vi "Test_RegisterForWrongType_Listbox_Error.vi"(8 "error in (no error)":errorcluster, 11 "TestActorEvents In":refnum<class "TestActorEvents.lvclass">) -> (0 "error out":errorcluster, 3 "TestActorEvents Out":refnum<class "TestActorEvents.lvclass">)   [LabVIEW 2017, in "TestActorEvents.lvlib" / "TestActorEvents.lvclass"]
uses:
  TestActorEvents.lvclass
  IViewModel/IViewModel/IViewModel.lvclass
  C:/Git/mva-framework/Framework/IViewManager/IViewManager/IViewManager.lvclass
  C:/Program Files (x86)/National Instruments/LabVIEW 2017/vi.lib/ActorFramework/Actor/Actor.lvclass
  ViewableListboxBadReg/ViewableListboxBadReg.lvclass
  C:/Git/mva-framework/_Test/Doubles/ViewableDoubles/LeakyViewable/LeakyViewable.lvclass
  C:/Git/mva-framework/Framework/IViewable/IViewable/IViewable.lvclass
  IModel/IModel/IModel.lvclass
  Mediator/Mediator/Mediator.lvclass
  C:/Git/mva-framework/Framework/IMediator/IMediator/IMediator.lvclass
  _Test/Doubles/ViewableDoubles/LeakyViewable/Leak Location.ctl
  _Test/Doubles/ViewableDoubles/LeakyViewable/LeakyViewable.lvclass/LeakyViewable.ctl
  IViewModel/IViewModel/IViewModel.lvclass/IViewModel.ctl
  IViewManager/IViewManager Messages/Launch Nested Views Msg/Launch Nested Views Msg.lvclass/Launch Nested Views Msg.ctl
  IViewManager/IViewManager/IViewManager.lvclass/IViewManager.ctl
  <vilib>/ActorFramework/Message Enqueuer/Message Enqueuer.lvclass/Message Enqueuer.ctl
  IViewManager/IViewManager Messages/Launch Nested Views Msg/Pack Launch Nested Views Msg.vi
  IViewManager/IViewManager/Write Startup Launch Nested Views Msg.vi
  <vilib>/ActorFramework/Message Enqueuer/Enqueue.vi
  <vilib>/ActorFramework/Stop Msg/Stop Msg.lvclass
  C:/Program Files (x86)/National Instruments/LabVIEW 2017/vi.lib/ActorFramework/Message/Message.lvclass
  <vilib>/ActorFramework/Message Priority Queue/Priority Enqueue.vi
  IViewable/IViewable/IViewable.lvclass
  IViewable/IApplicationStyle/IApplicationStyle.lvclass
  IViewManager/IViewManager Messages/Launch Nested Views Msg/Launch Nested Views Msg.lvclass
  <vilib>/addons/_JKI Toolkits/VI Tester/TestCase.llb/TestCase.lvclass
  <vilib>/ActorFramework/Actor/Actor.lvclass
  _Test/Doubles/ViewableDoubles/LeakyViewable/LeakyViewable.lvclass
  C:/Program Files (x86)/National Instruments/LabVIEW 2017/vi.lib/addons/_JKI Toolkits/VI Tester/TestCase.llb/TestCase.lvclass
panel:
  out "Error Status":errorcluster
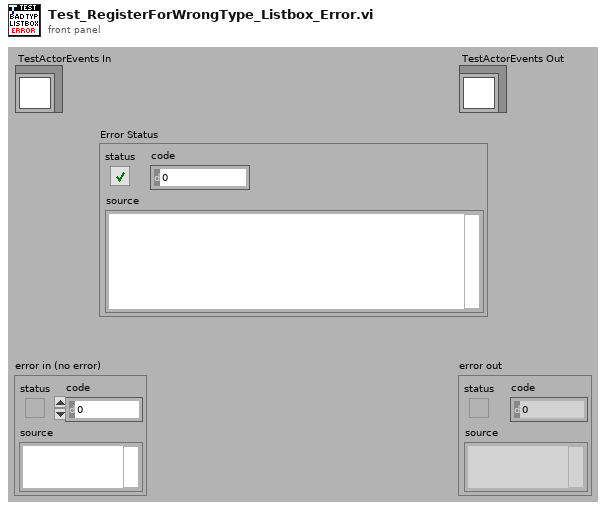
[diagram p1: front panel]
types:
  T1 = typedef "ViewableDoubles.lvlib/LeakyViewable.lvclass/Leak Location.ctl" = enum16{"Pre Launch Init", "Entering Actor Core", "Actor Core", "Exiting Actor Core", "Stop Core", "Handle Error"}
  T2 = cluster{"Location":T1, "State":refnum<class "IViewable.lvclass">, "Error Status":errorcluster}
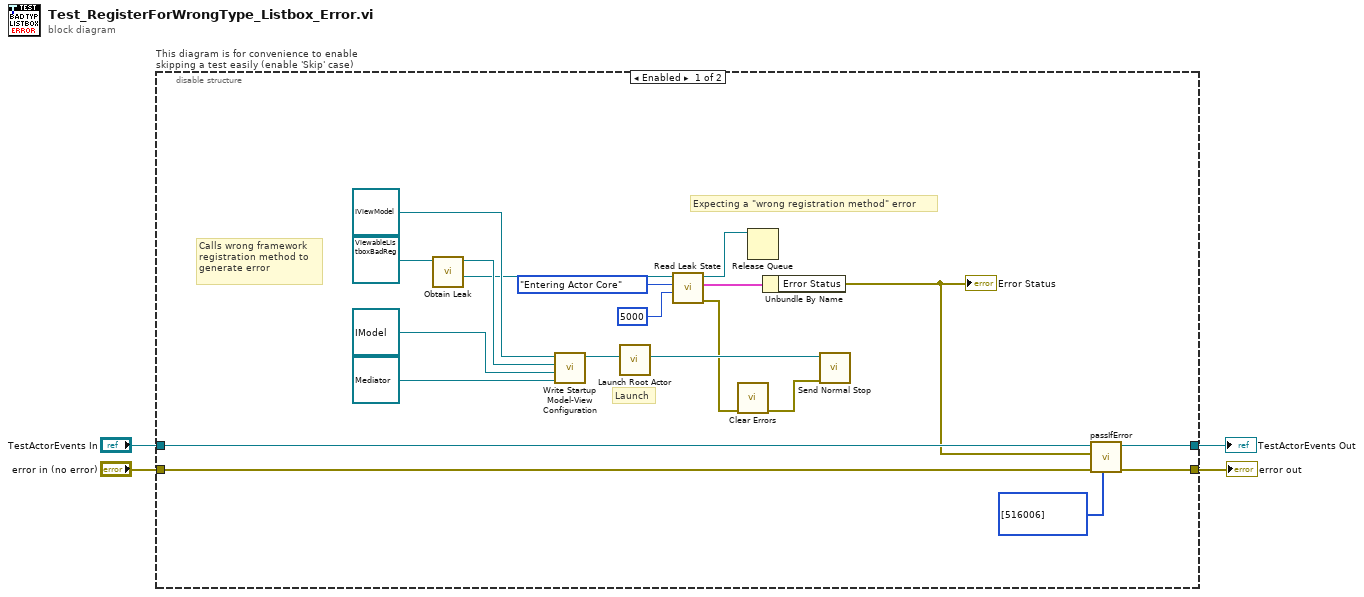
[diagram p0: block diagram]
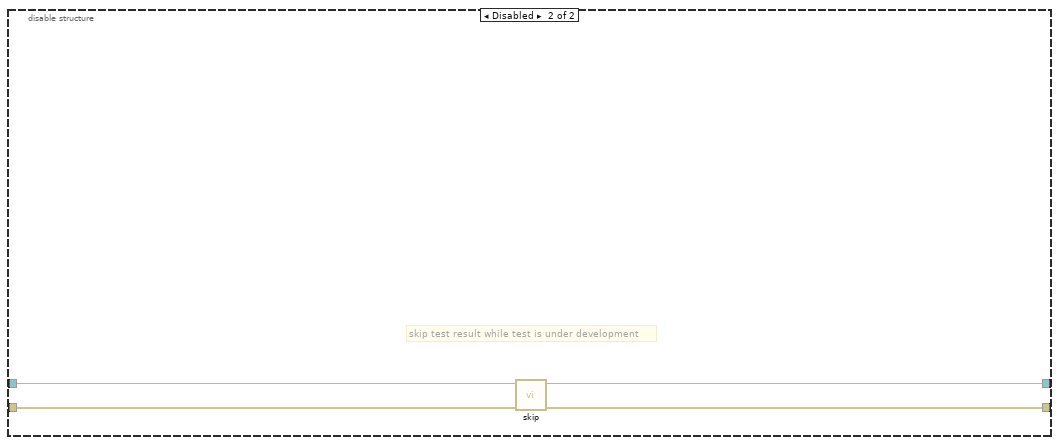
[diagram p2: hidden frame]
diagram:
  n1 = disable-structure "This diagram is for convenience to enable skipping a test easily (enable 'Skip' case)" shown="Enabled" {
    disable-tunnel: "TestActorEvents In" -> [w24 w28]
    disable-tunnel: [w23 w26] -> w1
    disable-tunnel: [w22 w27] -> w3
    disable-tunnel: "error in (no error)" -> [w21 w25]
    frame Enabled {
      # "Expecting a \"wrong registration method\" error"
      # "Calls wrong framework\nregistration method to\ngenerate error"
      # "Launch"
      n2 = call "Obtain Leak.vi"("LeakyViewable In"=refnum<class "ViewableListboxBadReg.lvclass"> refnum ("Startup View Configuration")) -> ("Viewable Leak Queue"=w13:refnum<queue>, "LeakyViewable Out"=w14:refnum<class "ViewableListboxBadReg.lvclass">)  [unwired: 9 in]
      n3 = call "Write Startup Model-View Configuration.vi"("Mediator Type"=refnum<class "Mediator.lvclass"> refnum ("Mediator"), "Model Type"=refnum<class "IModel.lvclass"> refnum ("Model"), "Startup View Configuration"=w14, "IViewModel In"=refnum<class "IViewModel.lvclass"> refnum) -> ("IViewModel Out"=w16:refnum<class "IViewModel.lvclass">)  [unwired: 7 in]
      n4 = call <vilib>:"Launch Root Actor.vi"("Actor"=w16) -> ("Actor's Enqueuer"=w8:refnum<class "Message Enqueuer.lvclass">)  [unwired: 9 in, 1 out]
      n5 = call "Read Leak State.vi"("timeout in ms (-1)"=5000, "Leak Location"=Leak_Location."Entering Actor Core", "Viewable Leak Queue In"=w13) -> ("error out"=w7:errorcluster, "State Snapshot"=w10:T2, "Viewable Leak Queue"=w5:refnum<queue>)  [unwired: 5 in, 1 out]
      n6 = call <vilib>:"Clear Errors.vi"("error in (no error)"=w7) -> ("error out"=w6:errorcluster)  [unwired: 5 in, 1 out]
      n7 = Release Queue(queue=w5) -> ()  [unwired: 2 in, 3 out]
      n8 = Unbundle By Name(w10) -> ("Error Status"=w9:errorcluster)
      "Error Status" <- w9
      n9 = call <vilib>:"Send Normal Stop.vi"("error in (no error)"=w6, "Message Enqueuer"=w8) -> ()  [unwired: 9 in, 1 out]
      n10 = call-dynamic "passIfError.vi"("passing error codes (default = any error code)"=i32[] [516006], "error in (no error)"=w21, "error"=w9, "TestCase in"=w24) -> ("error out"=w22:errorcluster, "TestCase out"=w23:refnum<class "TestActorEvents.lvclass">)  [unwired: 6 in]
    }
    frame Disabled {
      # "skip test result while test is under development"
      n11 = call <vilib>:"skip.vi"("error in (no error)"=w25, "TestCase in"=w28) -> ("error out"=w27:errorcluster, "TestCase out"=w26:refnum<class "TestActorEvents.lvclass">)  [unwired: 8 in]
    }
  }
  "error out" <- w3
  "TestActorEvents Out" <- w1
